vi "sv_Convert Phase.vi"(7 "phase units":enum16{"deg", "rad"}(ring), 8 "error in (no error)":errorcluster, 11 "phase lag [deg]":dbl format="%.2f") -> (0 "error out":errorcluster, 3 "converted phase lag":dbl format="%.3f", 5 "phase unit label":string)   [LabVIEW 2017, in "SoundVib_SingleTone.lvlib"]
uses:
  <vilib>/addons/Sound and Vibration/svt_Single Tone Measurements/SoundVib_SingleTone.lvlib
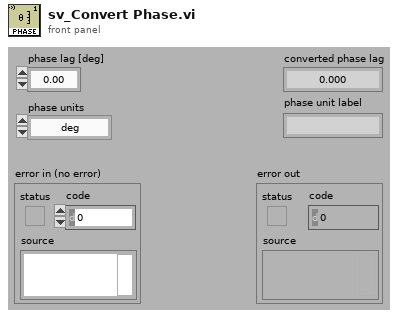
[diagram p1: front panel]
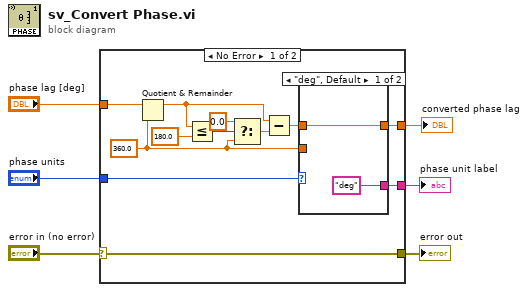
[diagram p0: block diagram]
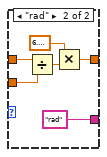
[diagram p2: hidden frame]
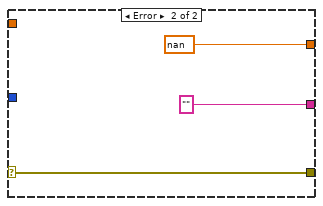
[diagram p3: hidden frame]
diagram:
  n1 = case shown="No Error" "error in (no error)" {
    selector: "error in (no error)" -> [w14 w29]
    tunnel: "phase lag [deg]" -> [w18 _]
    tunnel: "phase units" -> [w17 _]
    tunnel: [w16 nan] -> w4
    tunnel: [w15 "" ("phase unit label")] -> w3
    tunnel: [w14 w29] -> w1
    frame No Error {
      w11 = 360.0 ("y")
      n2 = Quotient & Remainder(x=w18, y=w11) -> (x-y*floor(x/y)=w7:dbl)  [unwired: 1 out]
      n3 = Less Or Equal?(x=w7, y=180.0) -> (x <= y?=w12:bool)
      n4 = Select(t=0.0, s=w12, f=w11) -> (s? t:f=w10:dbl)
      n5 = Subtract(x=w7, y=w10) -> (x-y=w13:dbl)
      n6 = case shown="\"deg\", Default" w17 {
        tunnel: [w20 w21] -> w16
        tunnel: w13 -> [w20 w25]
        tunnel: ["deg" ("phase unit label") "rad" ("phase unit label")] -> w15
        tunnel: w11 -> [_ w24]
        frame "deg", Default {
        }
        frame "rad" {
          n7 = Divide(x=w25, y=w24) -> (x/y=w23:dbl)
          n8 = Multiply(x=6.283185307179586, y=w23) -> (x*y=w21:dbl)
        }
      }
    }
    frame Error {
    }
  }
  "converted phase lag" <- w4
  "phase unit label" <- w3
  "error out" <- w1
